vi "Move to Position.vi"(8 "error in (no error)":errorcluster, 10 "Position":dbl[](array[numeric]), 11 "Stage Actor.lvlib:Stage.lvclass":refnum<class "Stage.lvclass">) -> (0 "error out":errorcluster, 3 "Actor out":refnum<class "Actor.lvclass">)   [LabVIEW 2018, in "Stage Actor.lvlib" / "Stage.lvclass"]
uses:
  Stage.lvclass
  <vilib>/ActorFramework/Actor/Actor.lvclass
  C:/Program Files/National Instruments/LabVIEW 2018/vi.lib/ActorFramework/Actor/Actor.lvclass
  Stage.lvclass/Stage.ctl
  <instrlib>/Zaber A Series/Zaber A Series.lvlib
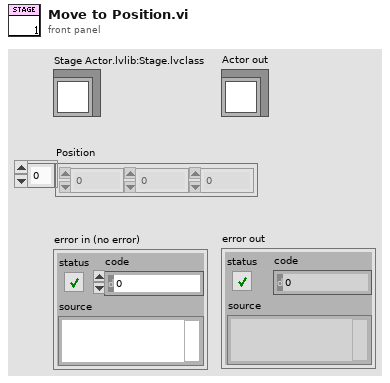
[diagram p1: front panel]
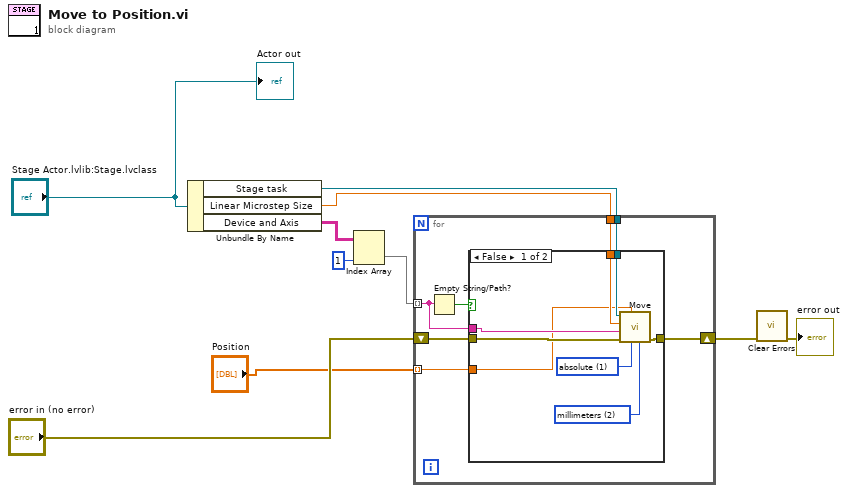
[diagram p0: block diagram]
diagram:
  n1 = Unbundle By Name("Stage Actor.lvlib:Stage.lvclass") -> ("Stage task"=w10:refnum<visa-resource-name>, "Linear Microstep Size"=w8:dbl, "Device and Axis"=w3:string[][])
  n2 = Index Array(array=w3, index (col)=1 ("disabled index (col)")) -> (element=w2:string[])  [unwired: 1 in]
  n3 = for {
    tunnel: w10 -> [w17]
    tunnel: w8 -> [w16]
    shift-right: [w14] -> w6
    shift-left: "error in (no error)" -> [w15]
    tunnel: w2 -> [w12] mode=indexing
    tunnel: "Position" -> [w11] mode=indexing
    n4 = Empty String/Path?(string/path=w12) -> (empty?=w13:bool)
    n5 = case shown="False" w13 {
      tunnel: w17 -> [w25 _]
      tunnel: w16 -> [w24 _]
      tunnel: w15 -> [w23 w26]
      tunnel: [w22 w26] -> w14
      tunnel: w12 -> [w19 _]
      tunnel: w11 -> [w18 _]
      frame False {
        w20 = u16 2 items=["microsteps", "microns", "millimeters", "inches", "degrees"] ("Units (0: microsteps)")
        w21 = u16 1 items=["relative", "absolute"] ("Movement Type (0: relative)")
        n6 = call <instrlib>:"Move.vi"("Units (0: microsteps)"=w20, "Movement Type (0: relative)"=w21, "Move Distance (0)"=w18, "error in (no error)"=w23, "Device and Axis"=w19, "Microstep Size (0)"=w24, "VISA resource name"=w25) -> ("error out"=w22:errorcluster)  [unwired: 3 in, 1 out]
      }
      frame True {
      }
    }
  }
  n7 = call <vilib>:"Clear Errors.vi"("error in (no error)"=w6) -> ("error out"=→"error out":errorcluster)  [unwired: 5 in, 1 out]
  "Actor out" <- "Stage Actor.lvlib:Stage.lvclass"
